vi "DS18B20 - convert raw temp.vi"(9 "MSB":u8 format="%.0x", 10 "LSB":u8 format="%.0x") -> (1 "Temp (C)":sgl, 2 "Temp (F)":sgl)   [LabVIEW 2014]
panel:
  # "Perform the temperature conversion for DS18B20\n- takes the raw 16 bit data coming from FPGA or LSB and MSB depending on boolean\n- calculates temperature in C and F"
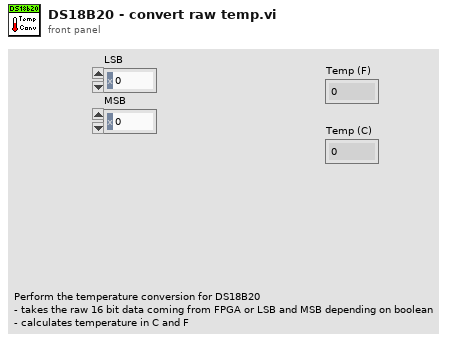
[diagram p1: front panel]
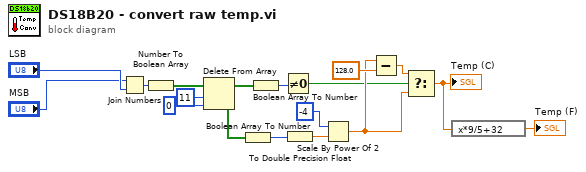
[diagram p0: block diagram]
diagram:
  n1 = Join Numbers(hi="MSB", lo="LSB") -> ((hi.lo)=w16:u16)
  n2 = Number To Boolean Array(number=w16) -> (Boolean array=w15:bool[])
  n3 = Delete From Array(array=w15, length=11, index=0) -> (deleted portion=w12:bool[], array with subset deleted=w7:bool[])
  n4 = Boolean Array To Number(Boolean array=w12) -> (number=w9:u16)
  n5 = Boolean Array To Number(Boolean array=w7) -> (number=w6:u8)
  n6 = Not Equal To 0?(x=w6) -> (x != 0?=w5:bool)
  n7 = To Double Precision Float(number=w9) -> (double precision float=w10:dbl)
  n8 = Scale By Power Of 2(n=-4, x=w10) -> (x*2^n=w8:dbl)
  n9 = Subtract(x=w8, y=128.0 ("x")) -> (x-y=w18:dbl)
  n10 = Select(t=w18, s=w5, f=w8) -> (s? t:f=w4:dbl)
  "Temp (C)" <- w4
  n11 = expression code="x*9/5+32"(w4) -> (→"Temp (F)":dbl)
